vi "Move Selected.vi"(8 "error in (no error)":errorcluster, 9 "target pos":dbl, 10 "Index":i32, 11 "VacuumLines in":refnum<class "VacuumLines.lvclass">) -> (0 "error out":errorcluster, 3 "VacuumLines out":refnum<class "VacuumLines.lvclass">)   [LabVIEW 2016, in "Hardware.lvlib" / "VacuumLine.lvlib" / "VacuumLines.lvclass"]
uses:
  <userlib>/Common Components/Hardware/Abstract System/VacuumLine/VacuumLines/VacuumLines.lvclass
  <userlib>/Common Components/Hardware/Abstract System/VacuumLine/VacuumLines/VacuumLines.lvclass/VacuumLines.ctl
  <userlib>/Common Components/Hardware/Abstract System/VacuumLine/VacuumLine/VacuumLine.lvclass
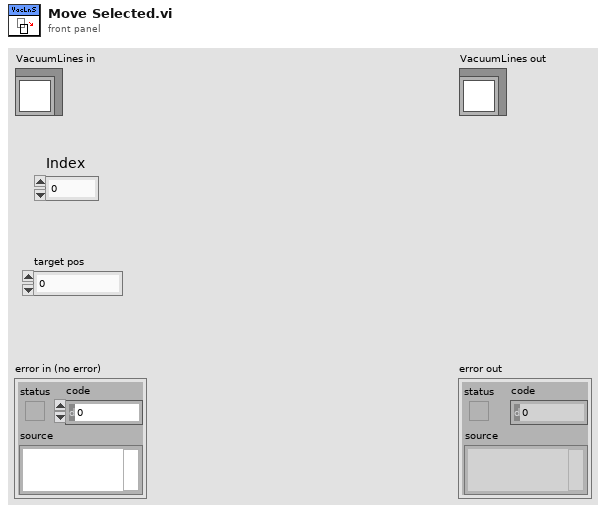
[diagram p1: front panel]
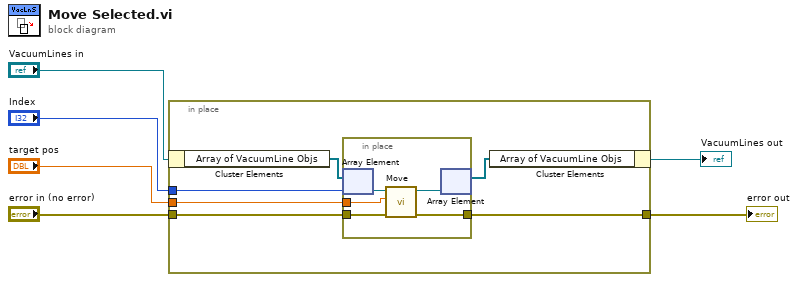
[diagram p0: block diagram]
diagram:
  n1 = in-place {
    in-place-border: "target pos" -> [w12]
    in-place-border: "Index" -> [w10]
    in-place-border: "error in (no error)" -> [w8]
    in-place-border: [w7] -> w1
    n2 = in-place-cluster #1("VacuumLines in") -> ("Array of VacuumLine Objs"=w11:refnum<class "VacuumLine.lvclass">[])
    n3 = in-place {
      in-place-border: w12 -> [w17]
      in-place-border: w8 -> [w15]
      in-place-border: [w14] -> w7
      n4 = in-place-array #2(w11, w10) -> (w13:refnum<class "VacuumLine.lvclass">)
      n5 = call <userlib>:"Move.vi"("error in (no error)"=w15, "target pos"=w17, "VacuumLine in"=w13) -> ("error out"=w14:errorcluster, "VacuumLine out"=w16:refnum<class "VacuumLine.lvclass">)  [unwired: 7 in]
      n6 = in-place-array #2(w16) -> (w9:refnum<class "VacuumLine.lvclass">[])  [unwired: 1 out]
    }
    n7 = in-place-cluster #1("Array of VacuumLine Objs"=w9) -> (→"VacuumLines out":refnum<class "VacuumLines.lvclass">)
  }
  "error out" <- w1
